vi "manageclick.vi"(0 "in":i8, 5 "total mine":i32, 7 "Button":u16, 9 "flag wrong in":i32, 12 "flag correct in":i32) -> (4 "out":i8, 10 "lose":bool=TRUE, 11 "flag wrong out":i32, 14 "flag correct out":i32, 15 "win1":bool=TRUE)   [LabVIEW 2025]
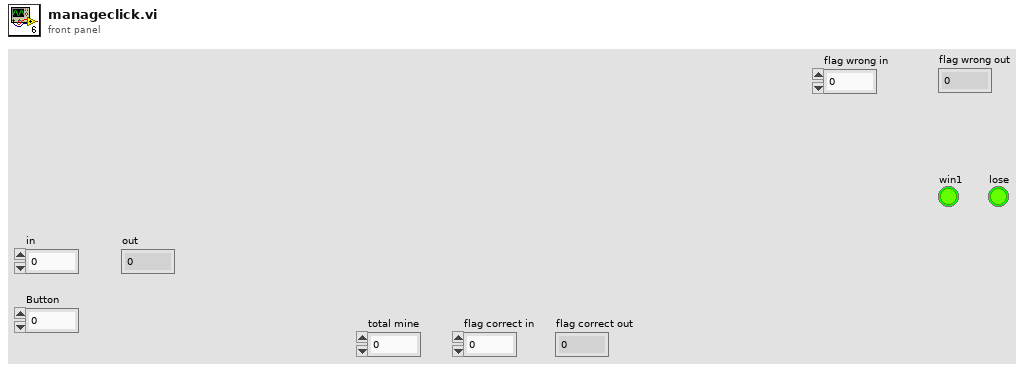
[diagram p1: front panel]
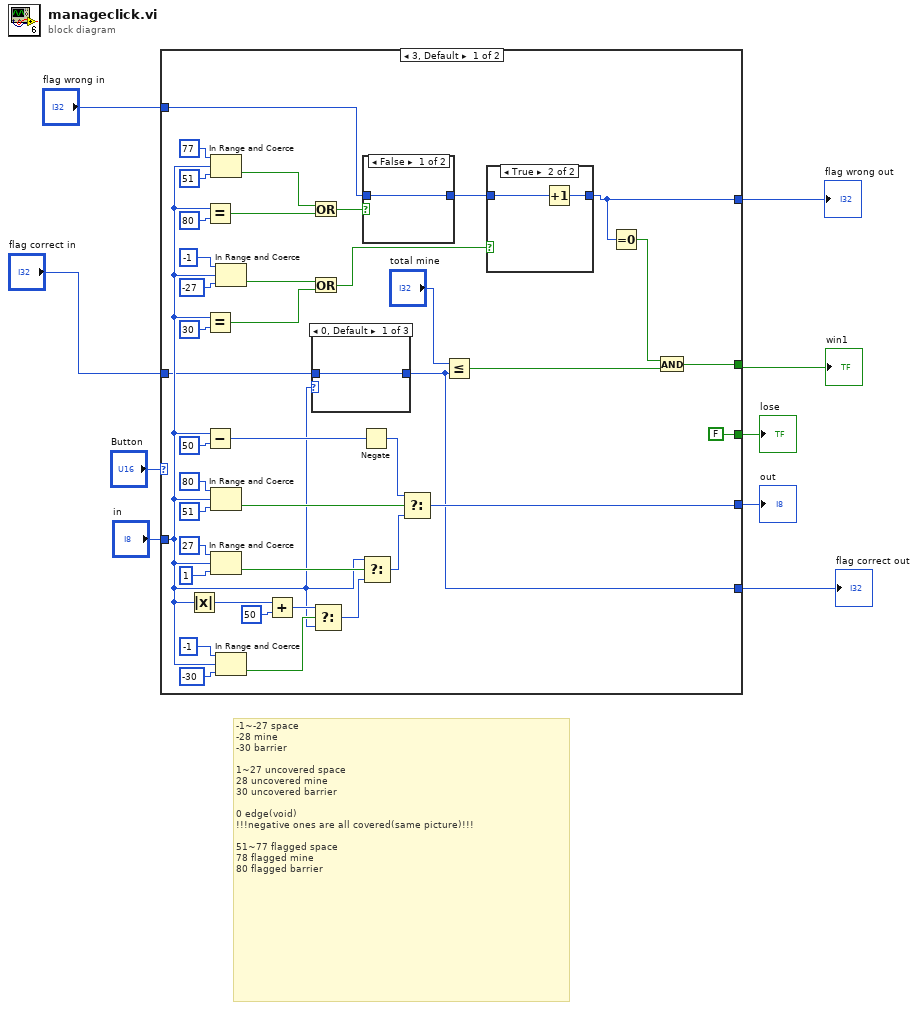
[diagram p0: block diagram]
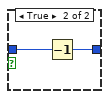
[diagram p2: hidden frame]
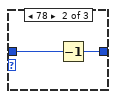
[diagram p4: hidden frame]
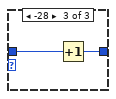
[diagram p5: hidden frame]
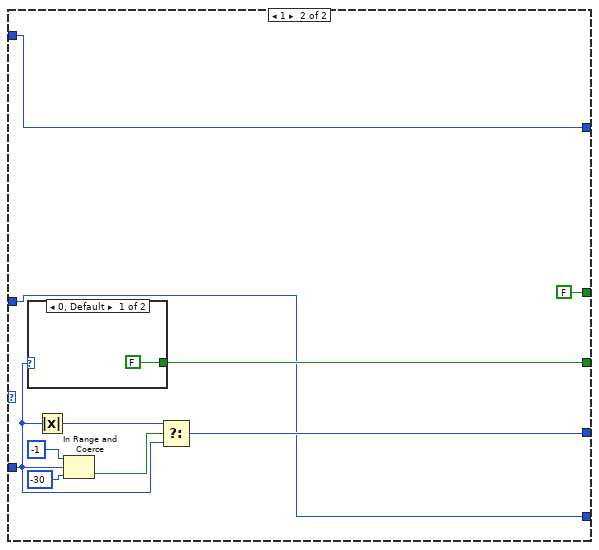
[diagram p6: hidden frame]
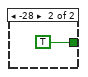
[diagram p7: hidden frame]
diagram:
  # "-1~-27 space\n-28 mine\n-30 barrier\n\n1~27 uncovered space\n28 uncovered mine\n30 uncovered barrier\n\n0 edge(void)\n!!!negative ones are all covered(same picture)!!!\n\n51~77 flagged space\n78 flagged mine\n80 flagged barrier"
  n1 = case shown="3, Default" "Button" {
    tunnel: "in" -> [w20 w65]
    tunnel: [w41 w67] -> w8
    tunnel: [w31 FALSE] -> w6
    tunnel: [FALSE ("lose") w64] -> w5
    tunnel: "flag wrong in" -> [w14 w63]
    tunnel: [w13 w63] -> w3
    tunnel: [w12 w62] -> w2
    tunnel: "flag correct in" -> [w10 w62]
    frame 3, Default {
      n2 = Absolute Value(x=w20) -> (abs(x)=w45:i8)
      n3 = Equal?(x=w20, y=i8 80) -> (x = y?=w17:bool)
      n4 = Equal?(x=w20, y=i8 30) -> (x = y?=w24:bool)
      n5 = Subtract(x=w20, y=i8 50) -> (x-y=w34:i8)
      n6 = In Range and Coerce(upper limit=i8 77, x=w20, lower limit=i8 51) -> (In Range?=w18:bool)  [unwired: 1 out]
      n7 = In Range and Coerce(upper limit=i8 80, x=w20, lower limit=i8 51) -> (In Range?=w48:bool)  [unwired: 1 out]
      n8 = In Range and Coerce(upper limit=i8 27, x=w20, lower limit=i8 1) -> (In Range?=w49:bool)  [unwired: 1 out]
      n9 = In Range and Coerce(upper limit=i8 -1, x=w20, lower limit=i8 -27) -> (In Range?=w25:bool)  [unwired: 1 out]
      n10 = In Range and Coerce(upper limit=i8 -1, x=w20, lower limit=i8 -30) -> (In Range?=w50:bool)  [unwired: 1 out]
      n11 = Add(x=w45, y=i8 50) -> (x+y=w43:i8)
      n12 = Or(x=w18, y=w17) -> (x .or. y?=w16:bool)
      n13 = Or(x=w25, y=w24) -> (x .or. y?=w23:bool)
      n14 = case shown="0, Default" w20 {
        tunnel: w10 -> [w57 w59 w61]
        tunnel: [w57 w58 w60] -> w12
        frame 0, Default {
        }
        frame 78 {
          n15 = Decrement(x=w59) -> (x-1=w58:i32)
        }
        frame -28 {
          n16 = Increment(x=w61) -> (x+1=w60:i32)
        }
      }
      n17 = Select(t=w43, s=w50, f=w20) -> (s? t:f=w38:i8)
      n18 = Negate(x=w34) -> (-x=w33:i8)
      n19 = Select(t=w20, s=w49, f=w38) -> (s? t:f=w42:i8)
      n20 = case shown="False" w16 {
        tunnel: w14 -> [w51 w53]
        tunnel: [w51 w52] -> w15
        frame False {
        }
        frame True {
          n21 = Decrement(x=w53) -> (x-1=w52:i32)
        }
      }
      n22 = Select(t=w33, s=w48, f=w42) -> (s? t:f=w41:i8)
      n23 = Less Or Equal?(x="total mine", y=w12) -> (x <= y?=w30:bool)
      n24 = case shown="True" w23 {
        tunnel: w15 -> [w54 w56]
        tunnel: [w54 w55] -> w13
        frame False {
        }
        frame True {
          n25 = Increment(x=w56) -> (x+1=w55:i32)
        }
      }
      n26 = Equal To 0?(x=w13) -> (x = 0?=w29:bool)
      n27 = And(x=w29, y=w30) -> (x .and. y?=w31:bool)
    }
    frame 1 {
      n28 = case shown="0, Default" w65 {
        tunnel: [FALSE ("lose") TRUE ("lose")] -> w64
        frame 0, Default {
        }
        frame -28 {
        }
      }
      n29 = Absolute Value(x=w65) -> (abs(x)=w71:i8)
      n30 = In Range and Coerce(upper limit=i8 -1, x=w65, lower limit=i8 -30) -> (In Range?=w68:bool)  [unwired: 1 out]
      n31 = Select(t=w71, s=w68, f=w65) -> (s? t:f=w67:i8)
    }
  }
  "out" <- w8
  "lose" <- w5
  "win1" <- w6
  "flag wrong out" <- w3
  "flag correct out" <- w2
